vi "TB-Options Dialog.vi"(0 "Parameters in":T4={"Low cutoff (kHz)"=0.0, "High cutoff (kHz)"=0.0, "Duration (min)"=0.0, "dB SPL"=100.0, "Waveform"=enum."Noise", "WAVfile"=path "", "refWav"=path "", "use mic correction"=FALSE, "micCorrFile"=path "", "Pistonphone Level (dB SPL)"=0.0, "Sampling rate (Hz)"=0.0, "Buffer length (s)"=0.0, "Stream mic"=FALSE, "Fine adjust"={"Max"=0.0, "Min"=0.0}, "Mic gain"=0.0, "atten"=0.0, "resol (Hz)"=0.0, "navgs"=0, "Allow Slack"=FALSE, "max starts"=0, "Freq (kHz)"=8.0, "Tma (s)"=0.0, "Streamed"=[], "Drive"=""}, 2 "Parent VI":refnum<vi>) -> (4 "Parameters out":T4={"Low cutoff (kHz)"=0.0, "High cutoff (kHz)"=0.0, "Duration (min)"=0.0, "dB SPL"=100.0, "Waveform"=enum."Noise", "WAVfile"=path "", "refWav"=path "", "use mic correction"=FALSE, "micCorrFile"=path "", "Pistonphone Level (dB SPL)"=0.0, "Sampling rate (Hz)"=0.0, "Buffer length (s)"=0.0, "Stream mic"=FALSE, "Fine adjust"={"Max"=0.0, "Min"=0.0}, "Mic gain"=0.0, "atten"=0.0, "resol (Hz)"=0.0, "navgs"=0, "Allow Slack"=FALSE, "max starts"=0, "Freq (kHz)"=8.0, "Tma (s)"=0.0, "Streamed"=[], "Drive"=""}, 8 "Canceled?":bool)   [LabVIEW 2020]
uses:
  Typedefs/TB-Parameters.ctl
  epl-vi-lib/Signal Synthesis VIs/Controls/Waveform XCtl/Waveform Enum.ctl
  epl-vi-lib/Utility VIs/Buttons/KCheckmarkBoolean 2.ctl
  epl-vi-lib/Utility VIs/Controls/KBackground Gradient/KBackground Gradient.xctl
  epl-vi-lib/Utility VIs/Slack VIs/Slack/Slack.xctl
  epl-vi-lib/Utility VIs/Controls/KTable/KTable.xctl
  Typedefs/TB-User.ctl
  epl-vi-lib/Connection VIs/Type Defs/Input sources.ctl
panel:
  in  "Tab":enum32{"Options", "Streaming", "Slack"}(tab)
  in  "max starts":i32 caption="Max number of starts (in case of error)"
  in  "Pistonphone Level":dbl caption="Pistonphone Level (dB SPL)"
  in  "Sampling rate (Hz)":dbl
  in  "Buffer length (s)":dbl
  in  "atten":dbl caption="Attenuation (dB)"
  in  "resol":dbl caption="Spectrum resolution (Hz)"
  in  "nspect":i32 caption="Spectrum averages"
  in  "Tma":dbl caption="Moving average (s)"
  out "Cal mic":u16(xcontrol) caption="Additional signals"
  in  "Table":u16(xcontrol) caption="Additional signals"
  in  "Stream raw data to disk":T1
  in  "Add Button":bool
  in  "Users":i32(listbox)
  in  "Slack":cluster{"config":T2, "users":T3[]}(xcontrol)
  in  "Gradient":dbl(xcontrol)
  in  "Cancel":bool
  in  "OK":bool
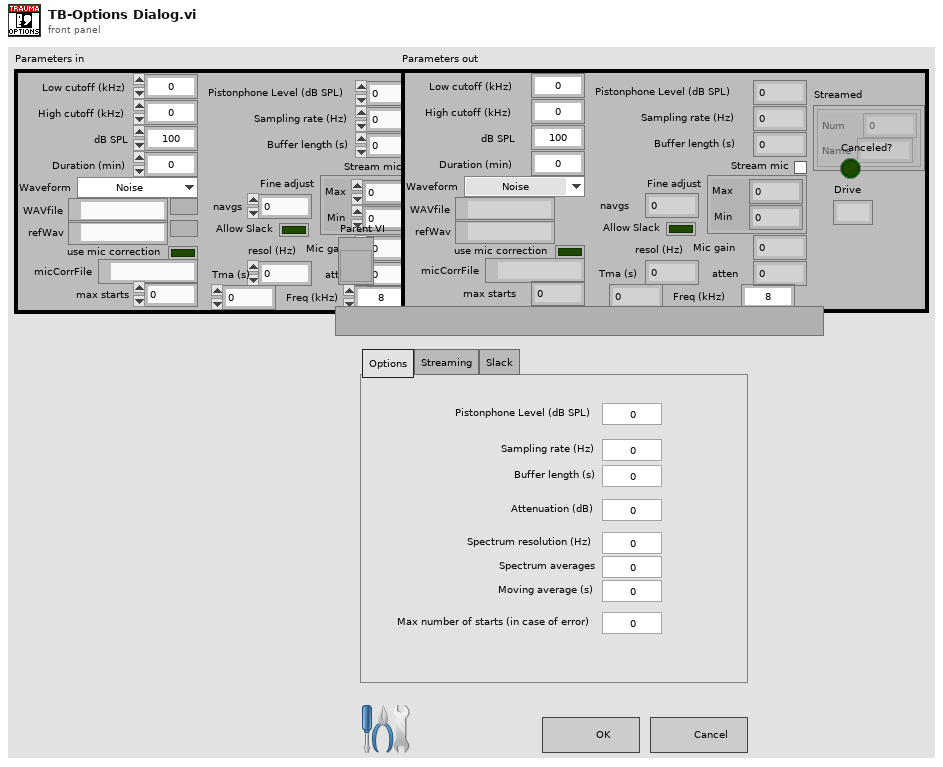
[diagram p1: front panel]
types:
  T1 = typedef "KCheckmarkBoolean 2.ctl" = bool
  T2 = typedef "Slack-Configuration.ctl" = cluster{"app_id":string, "authed_user":cluster{"id":string}, "access_token":string, "bot_user_id":string, "team":cluster{"id":string, "name":string}, "bot channel":cluster{"id":string, "name":string}, "bot_user_name":string}
  T3 = typedef "Slack-User.ctl" = cluster{"id":string, "name":string}
  T4 = typedef "TB-Parameters.ctl" = cluster{"Low cutoff (kHz)":dbl, "High cutoff (kHz)":dbl, "Duration (min)":dbl, "dB SPL":dbl, "Waveform":T5, "WAVfile":path, "refWav":path, "use mic correction":bool, "micCorrFile":path, "Pistonphone Level (dB SPL)":dbl, "Sampling rate (Hz)":dbl, "Buffer length (s)":dbl, "Stream mic":bool, "Fine adjust":cluster{"Max":dbl, "Min":dbl}, "Mic gain":dbl, "atten":dbl, "resol (Hz)":dbl, "navgs":i32, "Allow Slack":bool, "max starts":i32, "Freq (kHz)":dbl, "Tma (s)":dbl, "Streamed":cluster{"Num":i32, "Name":string}[], "Drive":string}
  T5 = typedef "Waveform Enum.ctl" = enum16{"OFF", "Tone", "Noise", "Pulse Train", "File", "FM Sweep", "Chirp Train", "Complex Tone", "FM Tone", "Moving Ripple"}
  T6 = typedef "TB-User.ctl" = cluster{"name":string, "id":string, "notify on errors":bool}
  T7 = enum8{"Enabled", "Disabled", "Disabled and Grayed Out"}
  T8 = typedef "Input sources.ctl" = u16
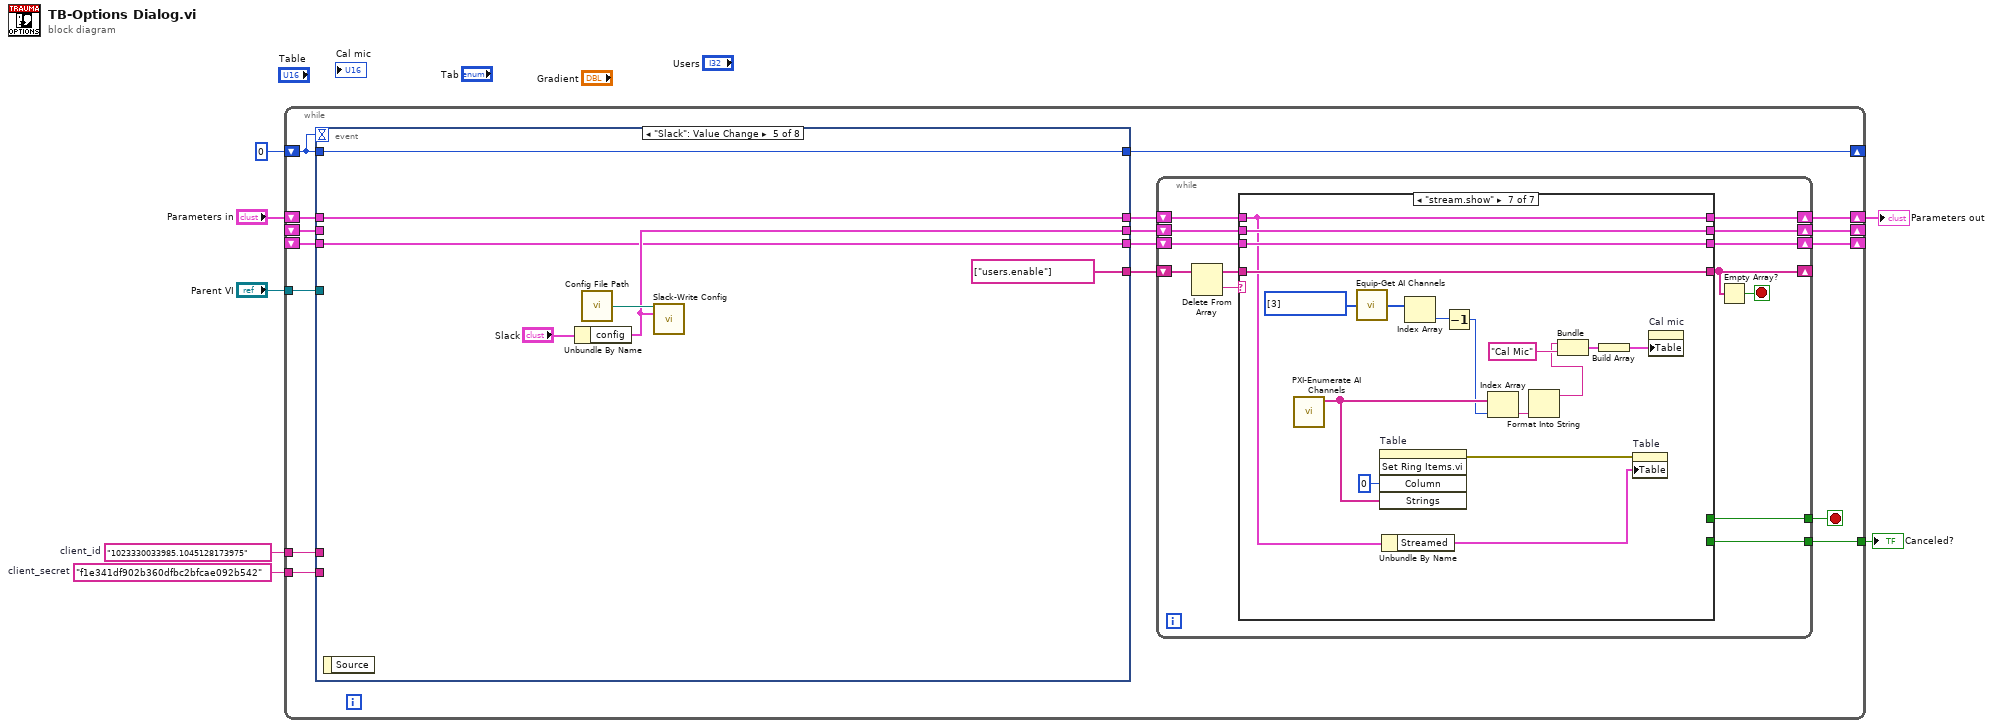
[diagram p0: block diagram]
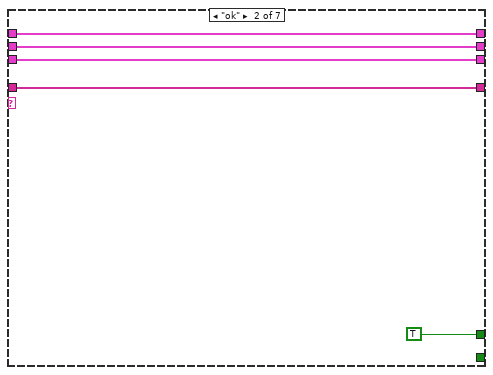
[diagram p3: hidden frame]
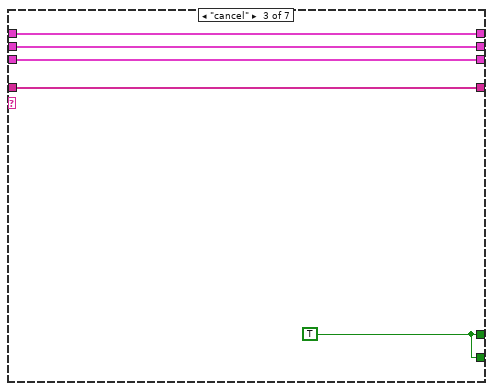
[diagram p4: hidden frame]
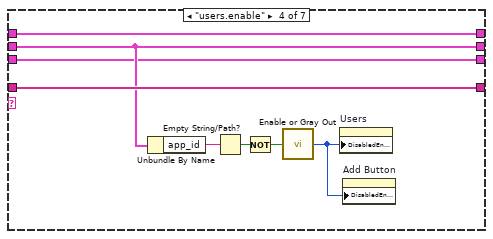
[diagram p5: hidden frame]
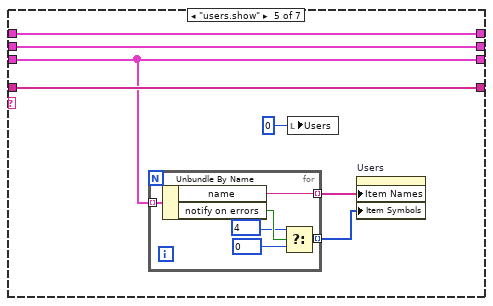
[diagram p6: hidden frame]
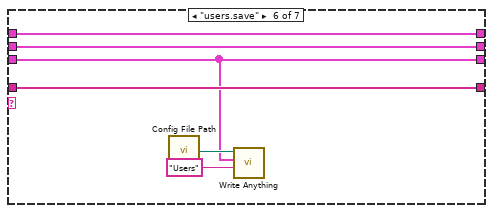
[diagram p7: hidden frame]
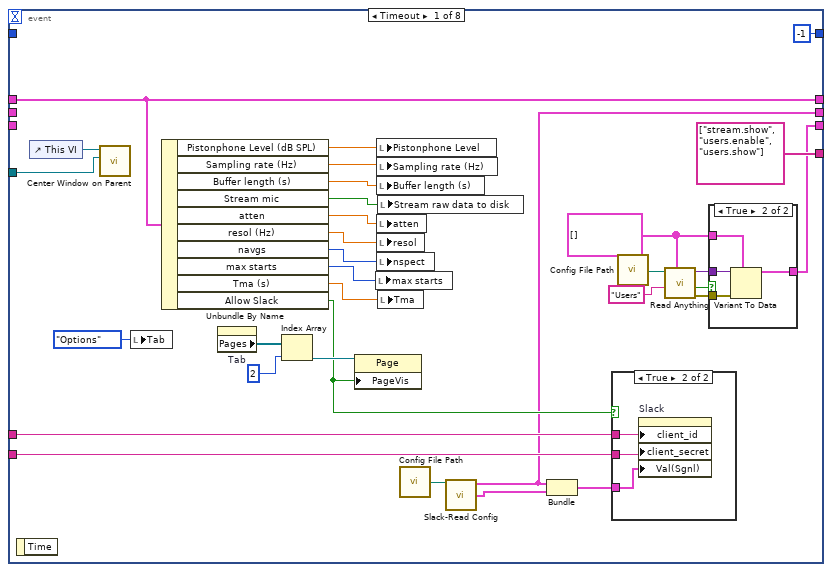
[diagram p8: hidden frame]
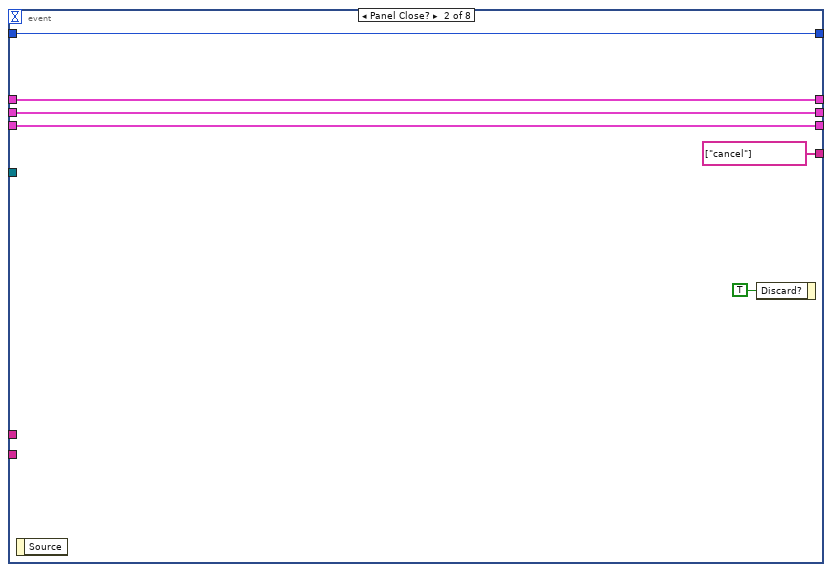
[diagram p11: hidden frame]
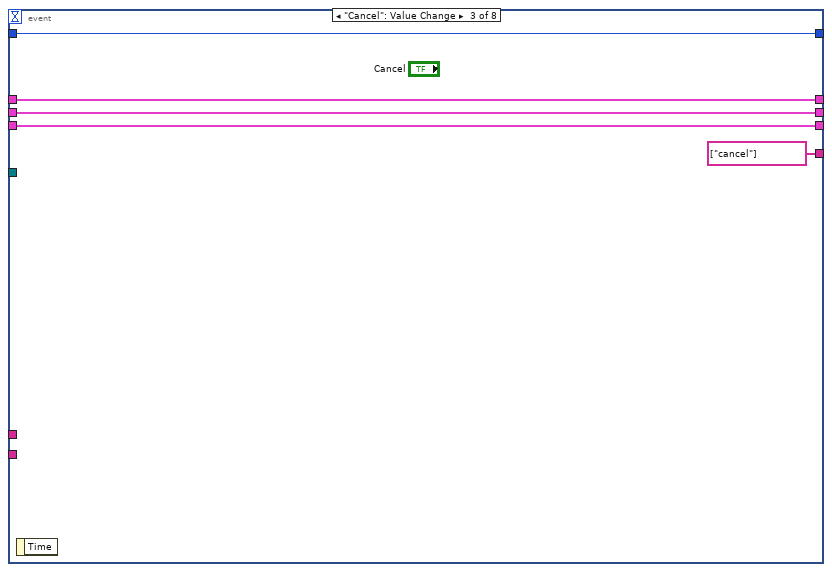
[diagram p12: hidden frame]
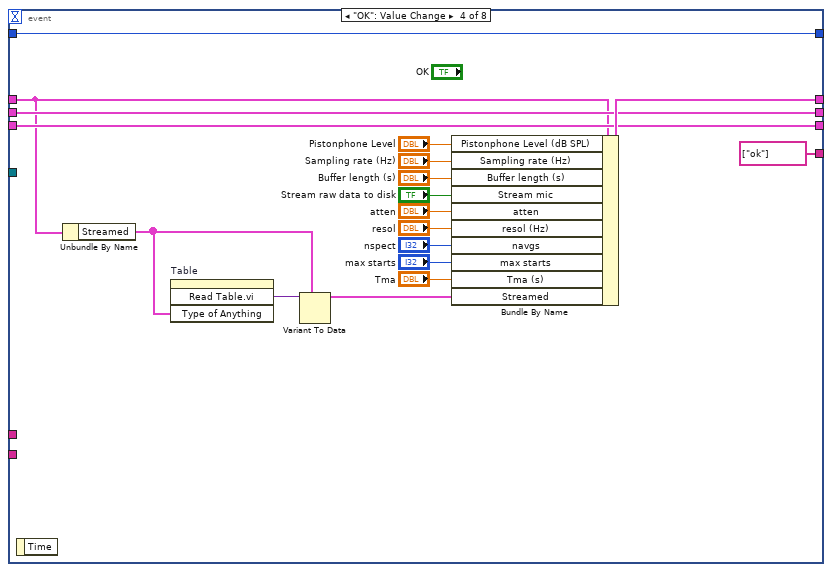
[diagram p13: hidden frame]
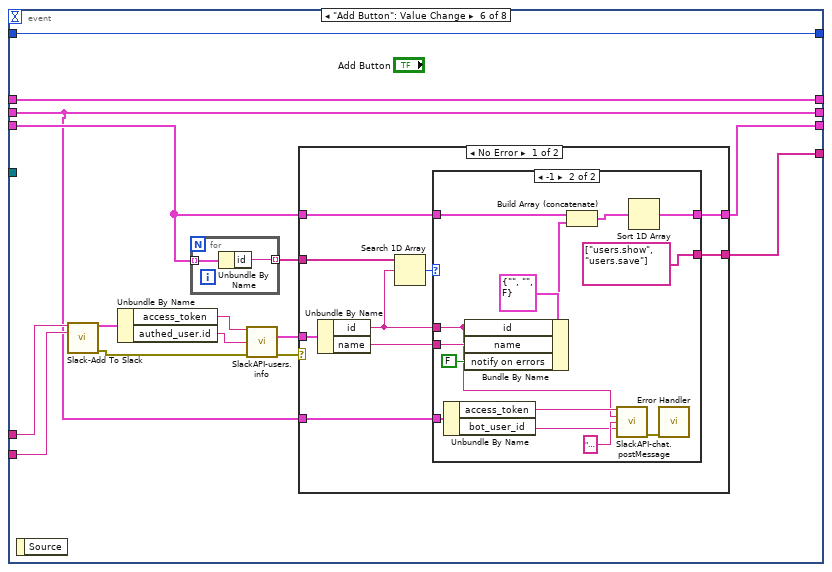
[diagram p14: hidden frame]
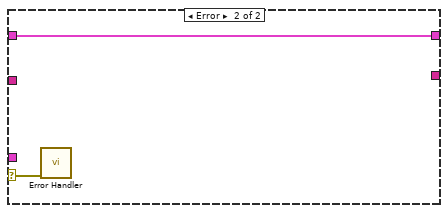
[diagram p16: hidden frame]
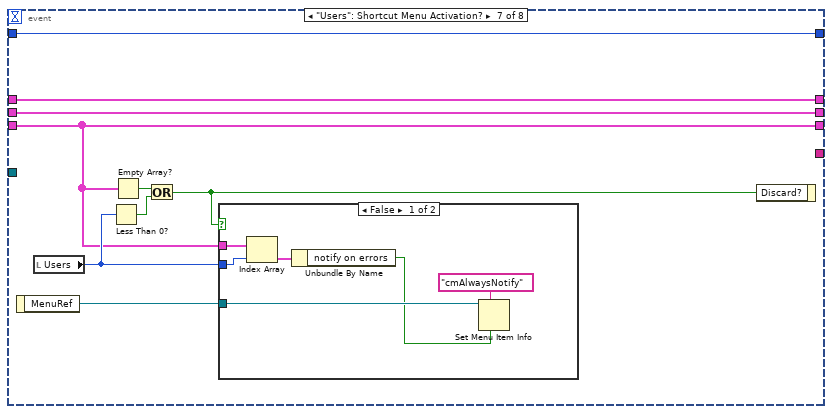
[diagram p17: hidden frame]
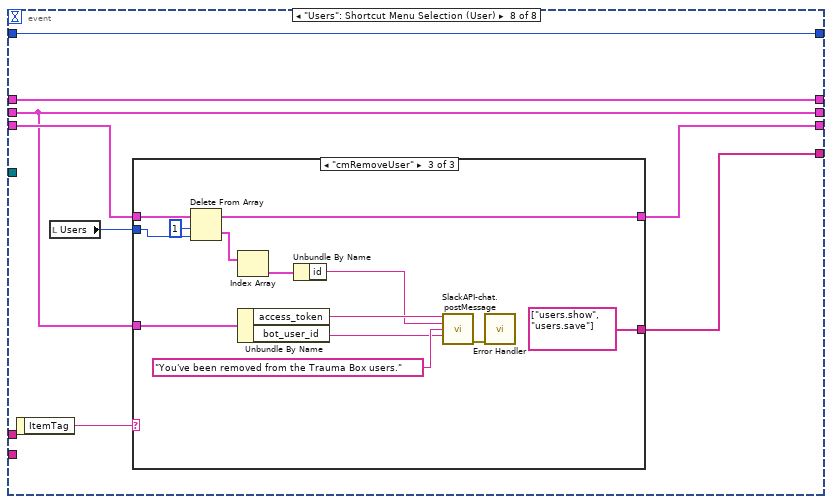
[diagram p19: hidden frame]
diagram:
  w1 = "f1e341df902b360dfbc2bfcae092b542"  # client_secret
  w2 = "1023330033985.1045128173975"  # client_id
  n1 = while {
    shift-right: [w24] -> _
    shift-left: 0 -> [w21]
    tunnel: [w11] -> w4
    shift-right: [w16] -> w5
    shift-left: "Parameters in" -> [w23]
    tunnel: "Parent VI" -> [w22]
    tunnel: w2 -> [w20]
    tunnel: w1 -> [w19]
    shift-right: [w14] -> _
    shift-left: _ -> [w13]
    shift-right: [w9] -> _
    shift-left: _ -> [w8]
    stop <- w12 stop-if-true
    n2 = event shown="[4] \"Slack\": Value Change" {
      selector: _ -> [_ _ _ _ _ _ _ _]
      dyn-events: _ -> [_ _ _ _ _ _ _ _]
      timeout: w21 -> [_ _ _ _ _ _ _ _]
      tunnel: [-1 w141 w146 w156 w170 w186 w223 w237] -> w24
      tunnel: w23 -> [w126 w140 w144 w150 w171 w185 w222 w236]
      tunnel: [w126 w140 w144 w164 w171 w185 w222 w236] -> w17
      tunnel: w22 -> [w117 _ _ _ _ _ _ _]
      tunnel: w21 -> [_ w141 w146 w156 w170 w186 w223 w237]
      tunnel: w20 -> [w108 _ _ _ _ w180 _ _]
      tunnel: w19 -> [w107 _ _ _ _ w179 _ _]
      tunnel: [w106 w139 w143 w153 w167 w172 w221 w230] -> w15
      tunnel: [string[] ["stream.show", "users.enable", "users.show"] string[] ["cancel"] string[] ["cancel"] string[] ["ok"] string[] ["users.enable"] w173 _ w231] -> w18
      tunnel: w13 -> [_ w139 w143 w153 _ w172 w221 w230]
      tunnel: [w99 w138 w142 w152 w165 w174 w216 w232] -> w10
      tunnel: w8 -> [_ w138 w142 w152 w165 w175 w216 w233]
      event Timeout {
        w100 = T6[] [] ("Array")
        n3 = event-data() -> ()  [unwired: 1 in, 1 out]
        n4 = control-ref of="This VI"() -> (w118:refnum<vi>)
        n5 = call "Center Window on Parent.vi"("Parent VI"=w117, "VI in"=w118) -> ()  [unwired: 8 in, 2 out]
        n6 = local write "Tab"(enum32{"Options", "Streaming", "Slack"}."Options" ("Tab")) -> ()
        n7 = Unbundle By Name(w126) -> ("Pistonphone Level (dB SPL)"=w125:dbl, "Sampling rate (Hz)"=w124:dbl, "Buffer length (s)"=w123:dbl, "Stream mic"=w122:bool, "atten"=w121:dbl, "resol (Hz)"=w120:dbl, "navgs"=w119:i32, "max starts"=w109:i32, "Tma (s)"=w97:dbl, "Allow Slack"=w111:bool)
        n8 = property on="Tab" class="TabCtl (strict)"() -> ("Pages"=w116:refnum<vi>[])  [unwired: 2 in, 2 out]
        n9 = Index Array(array=w116, index=2) -> (element=w114:refnum<vi>)
        n10 = property class="Page"(reference=w114, "PageVis"=w111) -> ()  [unwired: 1 in, 2 out]
        n11 = local write "max starts"(w109) -> ()
        n12 = local write "Pistonphone Level"(w125) -> ()
        n13 = local write "Sampling rate (Hz)"(w124) -> ()
        n14 = local write "Buffer length (s)"(w123) -> ()
        n15 = local write "atten"(w121) -> ()
        n16 = local write "resol"(w120) -> ()
        n17 = local write "nspect"(w119) -> ()
        n18 = local write "Stream raw data to disk"(w122) -> ()
        n19 = local write "Tma"(w97) -> ()
        n20 = call "Config File Path.vi"() -> ("Default config file name"=w113:path)  [unwired: 1 in]
        n21 = call "Slack-Read Config.vi"("AppName"=w113) -> ("config"=w106:T2, "users"=w110:T3[])  [unwired: 12 in, 1 out]
        n22 = Bundle("config"=w106, "users"=w110) -> (w112:cluster{"config":T2, "users":T3[]})  [unwired: 1 in]
        n23 = case shown="True" w111 {
          tunnel: w108 -> [_ w135]
          tunnel: w107 -> [_ w134]
          tunnel: w112 -> [_ w133]
          frame False {
          }
          frame True {
            n24 = property on="Slack" class="Slack (strict)"("client_id"=w135, "client_secret"=w134, "Val(Sgnl)"=w133) -> ()  [unwired: 2 in, 2 out]
          }
        }
        n25 = call "Config File Path.vi"() -> ("Default config file name"=w104:path)  [unwired: 1 in]
        n26 = call "Read Anything.vi"("Type of Anything"=w100, "Section Name (Name of \"Type of Anything\")"="Users" ("Section Name (Name of \"Anything\")"), "Path (dialog)"=w104) -> ("Error Out"=w101:errorcluster, "Found?"=w102:bool, "Anything"=w103:variant)  [unwired: 6 in]
        n27 = case shown="True" w102 {
          tunnel: w103 -> [_ w131]
          tunnel: w101 -> [_ w132]
          tunnel: w100 -> [w128 w130]
          tunnel: [w128 w129] -> w99
          frame False {
          }
          frame True {
            n28 = Variant To Data(error in=w132, type=w130, Variant=w131) -> (data=w129:T6[])  [unwired: 1 out]
          }
        }
      }
      event Panel Close? {
        n29 = event-data() -> ()  [unwired: 1 in, 1 out]
        n30 = event-data("Discard?"=TRUE) -> ()  [unwired: 1 in, 1 out]
      }
      event "Cancel": Value Change {
        n31 = event-data() -> ()  [unwired: 1 in, 1 out]
      }
      event "OK": Value Change {
        n32 = event-data() -> ()  [unwired: 1 in, 1 out]
        n33 = Unbundle By Name(w150) -> ("Streamed"=w148:cluster{"Num":i32, "Name":string}[])
        n34 = invoke on="Table" class="KTable (strict)" method="Read Table.vi"("Type of Anything"=w148) -> ("Read Table.vi"=w149:variant)  [unwired: 3 in, 3 out]
        n35 = Variant To Data(type=w148, Variant=w149) -> (data=w147:cluster{"Num":i32, "Name":string}[])  [unwired: 1 in, 1 out]
        n36 = Bundle By Name(cluster=w150, "Pistonphone Level (dB SPL)"="Pistonphone Level", "Sampling rate (Hz)"="Sampling rate (Hz)", "Buffer length (s)"="Buffer length (s)", "Stream mic"="Stream raw data to disk", "atten"="atten", "resol (Hz)"="resol", "navgs"="nspect", "max starts"="max starts", "Tma (s)"="Tma", "Streamed"=w147) -> (w164:T4)
      }
      event "Slack": Value Change {
        n37 = event-data() -> ()  [unwired: 1 in, 1 out]
        n38 = Unbundle By Name("Slack") -> ("config"=w167:T2)
        n39 = call "Config File Path.vi"() -> ("Default config file name"=w168:path)  [unwired: 1 in]
        n40 = call "Slack-Write Config.vi"("AppName"=w168, "config"=w167) -> ()  [unwired: 13 in, 1 out]
      }
      event "Add Button": Value Change {
        n41 = event-data() -> ()  [unwired: 1 in, 1 out]
        n42 = call "Slack-Add To Slack.vi"("client_id"=w180, "client_secret"=w179) -> ("config"=w181:T2, "error out"=w183:errorcluster)  [unwired: 12 in]
        n43 = Unbundle By Name(w181) -> ("access_token"=w182:string, "authed_user.id"=w184:string)
        n44 = for {
          tunnel: w175 -> [w188] mode=indexing
          tunnel: [w187] -> w176 mode=indexing
          n45 = Unbundle By Name(w188) -> ("id"=w187:string)
        }
        n46 = call "SlackAPI-users.info.vi"("token"=w182, "user"=w184, "error in (no error)"=w183) -> ("user"=w177:T3, "error out"=w178:errorcluster)  [unwired: 10 in, 1 out]
        n47 = case shown="No Error" w178 {
          selector: w178 -> [_ w213]
          tunnel: w177 -> [w197 _]
          tunnel: w176 -> [w195 _]
          tunnel: w175 -> [w192 w214]
          tunnel: [w191 w214] -> w174
          tunnel: [w190 _] -> w173
          tunnel: w172 -> [w189 _]
          frame No Error {
            n48 = Unbundle By Name(w197) -> ("id"=w194:string, "name"=w196:string)
            n49 = Search 1D Array(1D array=w195, element=w194) -> (index of element=w193:i32)  [unwired: 1 in]
            n50 = case shown="-1" w193 {
              tunnel: w196 -> [_ w211]
              tunnel: w194 -> [_ w200]
              tunnel: w192 -> [w198 w209]
              tunnel: [w198 w205] -> w191
              tunnel: [_ string[] ["users.show", "users.save"]] -> w190
              tunnel: w189 -> [_ w204]
              frame 0, Default {
              }
              frame -1 {
                n51 = Unbundle By Name(w204) -> ("access_token"=w203:string, "bot_user_id"=w201:string)
                n52 = Bundle By Name(cluster=T6 {"name"="", "id"="", "notify on errors"=FALSE} ("User"), "id"=w200, "name"=w211, "notify on errors"=FALSE ("always notify")) -> (w208:T6)
                n53 = Build Array (concatenate)(w209, w208) -> (w206:T6[])
                n54 = call "SlackAPI-chat.postMessage.vi"("access_token"=w203, "user ID"=w200, "message"="You've been added to the Trauma Box users.", "username"=w201) -> ("error out"=w199:errorcluster)  [unwired: 11 in]
                n55 = Sort 1D Array(array=w206) -> (sorted array=w205:T6[])
                n56 = call "Error Handler.vi"("error in (no error)"=w199) -> ()  [unwired: 13 in, 2 out]
              }
            }
          }
          frame Error {
            n57 = call "Error Handler.vi"("error in (no error)"=w213) -> ()  [unwired: 13 in, 2 out]
          }
        }
      }
      event "Users": Shortcut Menu Activation? {
        n58 = event-data() -> ("MenuRef"=w218:refnum<k9>)  [unwired: 1 in]
        n59 = local read "Users"() -> (w217:i32)
        n60 = Less Than 0?(x=w217) -> (x < 0?=w219:bool)
        n61 = Empty Array?(array=w216) -> (empty?=w220:bool)
        n62 = Or(x=w220, y=w219) -> (x .or. y?=w215:bool)
        n63 = case shown="False" w215 {
          tunnel: w218 -> [w226 _]
          tunnel: w217 -> [w228 _]
          tunnel: w216 -> [w229 _]
          frame False {
            n64 = Index Array(array=w229, index=w228) -> (element=w227:T6)
            n65 = Unbundle By Name(w227) -> ("notify on errors"=w224:bool)
            n66 = Set Menu Item Info(6:w224, 7:"cmAlwaysNotify" ("item tag"), 11:w226) -> ()  [unwired: 4 in, 2 out]
          }
          frame True {
          }
        }
        n67 = event-data("Discard?"=w215) -> ()  [unwired: 1 in, 1 out]
      }
      event "Users": Shortcut Menu Selection (User) {
        n68 = event-data() -> ("ItemTag"=w235:string)  [unwired: 1 in]
        n69 = local read "Users"() -> (w234:i32)
        n70 = case shown="\"cmRemoveUser\"" w235 {
          tunnel: w233 -> [w238 w243 w258]
          tunnel: w234 -> [_ w241 w257]
          tunnel: [w238 w240 w255] -> w232
          tunnel: [_ string[] ["users.show", "users.save"] string[] ["users.show", "users.save"]] -> w231
          tunnel: w230 -> [_ _ w250]
          frame "", Default {
          }
          frame "cmAlwaysNotify" {
            n71 = Index Array(array=w243, index=w241) -> (element=w245:T6)
            n72 = Unbundle By Name(w245) -> ("notify on errors"=w246:bool)
            n73 = Not(x=w246) -> (.not. x?=w244:bool)
            n74 = Bundle By Name(cluster=w245, "notify on errors"=w244) -> (w242:T6)
            n75 = Replace Array Subset(array=w243, new element=w242, index=w241) -> (w240:T6[])
          }
          frame "cmRemoveUser" {
            n76 = Delete From Array(array=w258, length=1, index=w257) -> (deleted portion=w249:T6[], array with subset deleted=w255:T6[])
            n77 = Index Array(array=w249) -> (element=w248:T6)  [unwired: 1 in]
            n78 = Unbundle By Name(w250) -> ("access_token"=w254:string, "bot_user_id"=w252:string)
            n79 = Unbundle By Name(w248) -> ("id"=w247:string)
            n80 = call "SlackAPI-chat.postMessage.vi"("access_token"=w254, "user ID"=w247, "message"="You've been removed from the Trauma Box users.", "username"=w252) -> ("error out"=w251:errorcluster)  [unwired: 11 in]
            n81 = call "Error Handler.vi"("error in (no error)"=w251) -> ()  [unwired: 13 in, 2 out]
          }
        }
      }
    }
    n82 = while {
      shift-right: [w34] -> _
      shift-left: w18 -> [w37]
      shift-right: [w31] -> w16
      shift-left: w17 -> [w32]
      shift-right: [w29] -> w14
      shift-left: w15 -> [w30]
      tunnel: [w28] -> w12
      tunnel: [w27] -> w11
      shift-right: [w25] -> w9
      shift-left: w10 -> [w26]
      stop <- w33 stop-if-true
      n83 = Delete From Array(array=w37) -> (deleted portion=w35:string, array with subset deleted=w36:string[])  [unwired: 2 in]
      n84 = case shown="\"stream.show\"" w35 {
        tunnel: w36 -> [w41 w46 w51 w59 w66 w78 w95]
        tunnel: [w41 w46 w51 w59 w66 w78 w95] -> w34
        tunnel: w32 -> [w40 w45 w50 w58 w65 w77 w80]
        tunnel: [w40 w45 w50 w58 w65 w77 w80] -> w31
        tunnel: w30 -> [w39 w44 w49 w57 w64 w76 w94]
        tunnel: [w39 w44 w49 w57 w64 w76 w94] -> w29
        tunnel: [_ TRUE w48 _ _ _ _] -> w28
        tunnel: [_ _ w48 _ _ _ _] -> w27
        tunnel: w26 -> [w38 w42 w47 w52 w63 w74 w93]
        tunnel: [w38 w42 w47 w52 w63 w74 w93] -> w25
        frame "", Default {
        }
        frame "ok" {
        }
        frame "cancel" {
          w48 = TRUE
        }
        frame "users.enable" {
          n85 = Unbundle By Name(w57) -> ("app_id"=w56:string)
          n86 = Empty String/Path?(string/path=w56) -> (empty?=w55:bool)
          n87 = Not(x=w55) -> (.not. x?=w54:bool)
          n88 = call "Enable or Gray Out.vi"("Boolean"=w54) -> ("Disabled"=w53:T7)
          n89 = property on="Users" class="LstBox (strict)"("DisabledEnum"=w53) -> ()  [unwired: 2 in, 2 out]
          n90 = property on="Add Button" class="Bool"("DisabledEnum"=w53) -> ()  [unwired: 2 in, 2 out]
        }
        frame "users.show" {
          n91 = for {
            tunnel: w63 -> [w72] mode=indexing
            tunnel: [w71] -> w62 mode=indexing
            tunnel: [w68] -> w60 mode=indexing
            n92 = Unbundle By Name(w72) -> ("name"=w71:string, "notify on errors"=w70:bool)
            n93 = Select(t=4, s=w70, f=0) -> (s? t:f=w68:i32)
          }
          n94 = local write "Users"(0) -> ()
          n95 = property on="Users" class="LstBox (strict)"("Item Names"=w62, "Item Symbols"=w60) -> ()  [unwired: 2 in, 2 out]
        }
        frame "users.save" {
          n96 = call "Config File Path.vi"() -> ("Default config file name"=w75:path)  [unwired: 1 in]
          n97 = call "Write Anything.vi"("Section Name (Name of \"Anything\")"="Users" ("Section Name (Name of \"Anything\")"), "Anything"=w74, "Path (dialog)"=w75) -> ()  [unwired: 7 in, 2 out]
        }
        frame "stream.show" {
          w91 = T8[] [3] items=["--unused--", "Probe Mic Right", "Probe Mic Left", "Cal Mic", "ABR", "CAP Right", "CAP Left", "Startle piezo", "Temperature", "Heart rate", "Accelerometer", "Startle piezo 2"] ("Inputs")
          n98 = call "PXI-Enumerate AI Channels.vi"() -> ("AI.PhysicalChans"=w85:tag[])  [unwired: 11 in]
          n99 = call "Equip-Get AI Channels.vi"("Inputs"=w91) -> ("AI Channels"=w90:i32[])  [unwired: 13 in, 1 out]
          n100 = invoke on="Table" class="KTable (strict)" method="Set Ring Items.vi"("Column"=0, "Strings"=w85) -> (error out=w81:errorcluster)  [unwired: 3 in, 4 out]
          n101 = Unbundle By Name(w80) -> ("Streamed"=w79:cluster{"Num":i32, "Name":string}[])
          n102 = Index Array(array=w90) -> (element=w89:i32)  [unwired: 1 in]
          n103 = Decrement(x=w89) -> (x-1=w84:i32)
          n104 = Index Array(array=w85, index=w84) -> (element=w83:tag)
          n105 = Format Into String(w83) -> (resulting string=w82:string)  [unwired: 3 in, 1 out]
          n106 = Bundle(w82, "Cal Mic") -> (w87:cluster{string, string})  [unwired: 1 in]
          n107 = Build Array(w87) -> (w86:cluster{string, string}[])
          n108 = property on="Table" class="KTable (strict)"(error in=w81, "Table"=w79) -> ()  [unwired: 1 in, 2 out]
          n109 = property on="Cal mic" class="KTable (strict)"("Table"=w86) -> ()  [unwired: 2 in, 2 out]
        }
      }
      n110 = Empty Array?(array=w34) -> (empty?=w33:bool)
    }
  }
  "Parameters out" <- w5
  "Canceled?" <- w4
